vi "Read write operation timeout.vi"(8 "error in (no error)":errorcluster, 11 "Socket in":refnum<class "WebSocket.lvclass">) -> (0 "error out":errorcluster, 2 "write operation timeout":i32=10000, 3 "Socket out":refnum<class "WebSocket.lvclass">)   [LabVIEW 2021, in "WebSockets.lvlib" / "WebSocket.lvclass"]
uses:
  WebSocket.lvclass
  WebSocket.lvclass/WebSocket.ctl
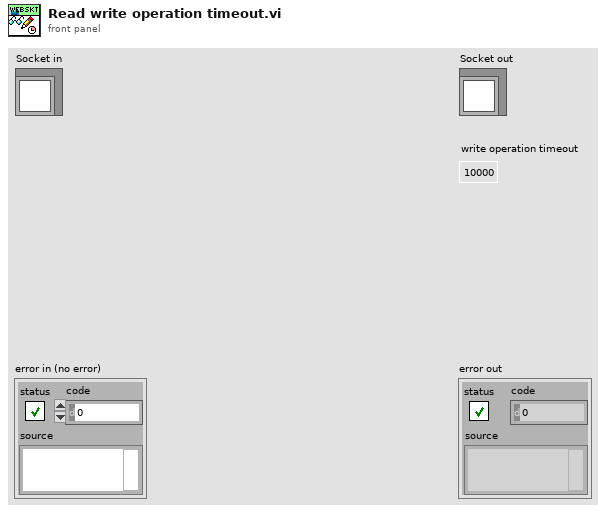
[diagram p1: front panel]
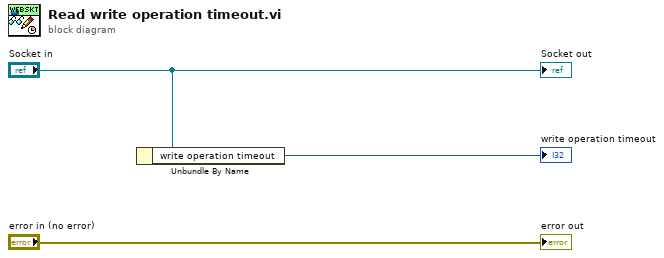
[diagram p0: block diagram]
diagram:
  n1 = Unbundle By Name("Socket in") -> ("write operation timeout"=→"write operation timeout":i32)
  "error out" <- "error in (no error)"
  "Socket out" <- "Socket in"
